vi "Channel Info.vi"(8 "error in":errorcluster, 11 "Input Channels in":refnum<class "Input Channels.lvclass">) -> (0 "error out":errorcluster, 1 "Channel Active?":bool, 2 "Channel Information":T1={"Channel Direction"=enum."Module Output", "Alias"="", "Refresh (ms)"=1000.0, "Scaling Information"={"Active"=FALSE, "Scaling Type"=enum."Linear", "Output Minimum"=0.0, "Output Maximum"=1.0, "Raw Minimum"=0.0, "Raw Maximum"=1.0, "Output Unit"="", "Function"="", "Lookup Table"=""}, "Value Type"=enum."double", "Subchannels"=[], "Auxiliary Data"=variant, "Group"=-1}, 3 "Input Channels out":refnum<class "Input Channels.lvclass">)   [LabVIEW 2020, in "Plugin.lvlib" / "Input Channels.lvclass"]
doc: "Reads the input channel data and updates the channel information cluster."
uses:
  Input Channels.lvclass
  C:/SVN_LabSys/labsys_lvcode/LabSys_SourceCode/Plugin Template/Source/Code/Channels/Plugin_Channels.lvclass
  builds/Libraries/LabSys Framework.lvlibp/Configuration Storage/Test Configuration/Channel Information.ctl
  builds/Libraries/LabSys Framework.lvlibp/Configuration Storage/Test Configuration/Channel Directions.ctl
  builds/Libraries/LabSys Framework.lvlibp/Configuration Storage/Test Configuration/Scaling Information.ctl
  builds/Libraries/LabSys Framework.lvlibp/Configuration Storage/Test Configuration/Scaling Types.ctl
  builds/Libraries/Framework Base Library.lvlibp/Value Types.ctl
  builds/Libraries/LabSys Framework.lvlibp/Configuration Storage/Test Configuration/Subchannel Information.ctl
  Typedefs/Channel Type.ctl
  UI_Class/Auxiliary Data.ctl
  Plugin_Channels.lvclass
  builds/Libraries/Framework Base Library.lvlibp
  builds/Libraries/LabSys Framework.lvlibp/Configuration Storage/Test Configuration/Test Configuration.lvclass
  UI_Class/Plugin_UI.lvclass
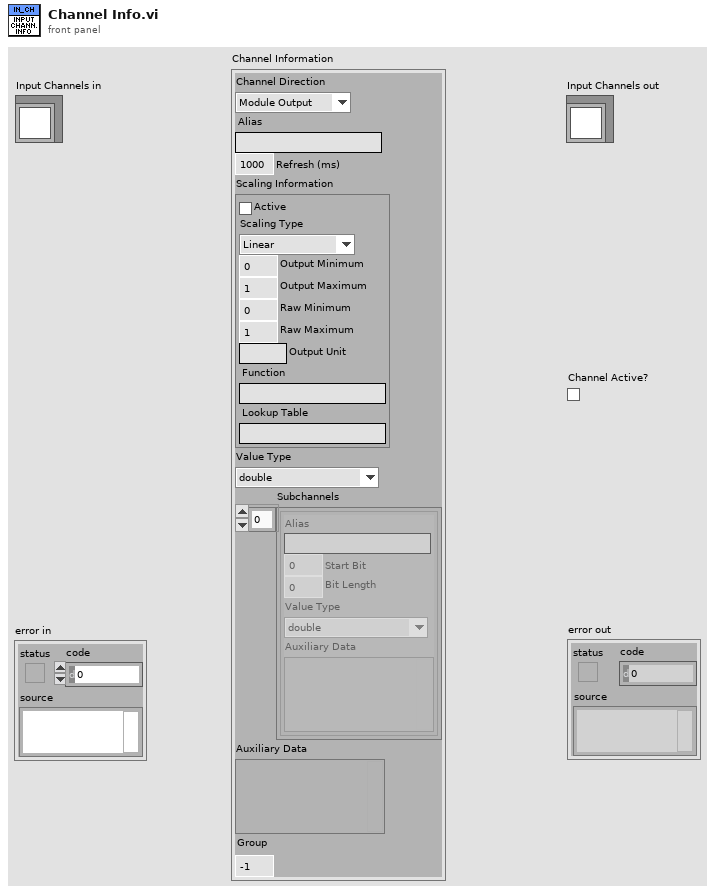
[diagram p1: front panel]
types:
  T1 = typedef "LabSys Framework.lvlibp/Configuration Storage.lvlib/Test Configuration.lvclass/Channel Information.ctl" = cluster{"Channel Direction":T2, "Alias":string, "Refresh (ms)":dbl, "Scaling Information":T3, "Value Type":T5, "Subchannels":T6[], "Auxiliary Data":variant, "Group":i32}
  T2 = typedef "LabSys Framework.lvlibp/Configuration Storage.lvlib/Test Configuration.lvclass/Channel Directions.ctl" = enum8{"Module Input", "Module Output"}
  T3 = typedef "LabSys Framework.lvlibp/Configuration Storage.lvlib/Test Configuration.lvclass/Scaling Information.ctl" = cluster{"Active":bool, "Scaling Type":T4, "Output Minimum":dbl, "Output Maximum":dbl, "Raw Minimum":dbl, "Raw Maximum":dbl, "Output Unit":string, "Function":string, "Lookup Table":string}
  T4 = typedef "LabSys Framework.lvlibp/Configuration Storage.lvlib/Test Configuration.lvclass/Scaling Types.ctl" = enum8{"Linear", "Function", "Lookup Table"}
  T5 = typedef "Framework Base Library.lvlibp/Value Types.ctl" = enum8{"Unknown", "double", "double array", "Waveform", "DigWaveform", "Boolean", "Decimal", "String", "Db2Message", "Byte Array", "Unsigned Decimal"}
  T6 = typedef "LabSys Framework.lvlibp/Configuration Storage.lvlib/Test Configuration.lvclass/Subchannel Information.ctl" = cluster{"Alias":string, "Start Bit":u32, "Bit Length":u32, "Value Type":T5, "Auxiliary Data":variant}
  T7 = typedef "Plugin.lvlib/Plugin_UI.lvclass/Auxiliary Data.ctl" = cluster{"Plugin_Data":refnum<class "Plugin_Channels.lvclass">}
  T8 = typedef "Plugin.lvlib/Plugin_Channels.lvclass/Channel Type.ctl" = enum16{"Input", "Output"}
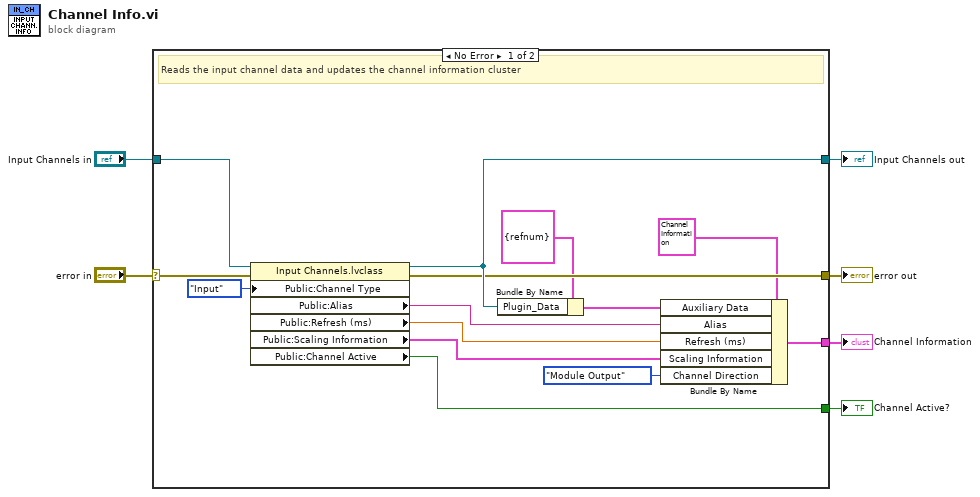
[diagram p0: block diagram]
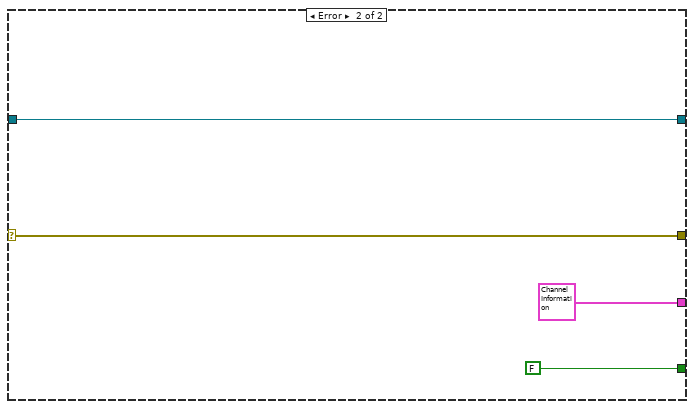
[diagram p2: hidden frame]
diagram:
  n1 = case shown="No Error" "error in" {
    selector: "error in" -> [w20 w24]
    tunnel: [w15 w24] -> w5
    tunnel: [w16 w23] -> w3
    tunnel: "Input Channels in" -> [w17 w23]
    tunnel: [w11 FALSE ("Public:Channel Active")] -> w2
    tunnel: [w10 T1 {"Channel Direction"=enum."Module Output", "Alias"="", "Refresh (ms)"=1000.0, "Scaling Information"={"Active"=FALSE, "Scaling Type"=enum."Linear", "Output Minimum"=0.0, "Output Maximum"=1.0, "Raw Minimum"=0.0, "Raw Maximum"=1.0, "Output Unit"="", "Function"="", "Lookup Table"=""}, "Value Type"=enum."double", "Subchannels"=[], "Auxiliary Data"=variant, "Group"=-1} ("Channel Information")] -> w1
    frame No Error {
      # "Reads the input channel data and updates the channel information cluster"
      n2 = property class="Input Channels.lvclass"(reference=w17, error in=w20, "Public:Channel Type"=Channel_Type."Input" ("Channel Type")) -> (reference out=w16:refnum<class "Input Channels.lvclass">, error out=w15:errorcluster, "Public:Alias"=w14:string, "Public:Refresh (ms)"=w13:dbl, "Public:Scaling Information"=w12:T3, "Public:Channel Active"=w11:bool)
      n3 = Bundle By Name(cluster=T7 {"Plugin_Data"=refnum} ("Auxiliary Data"), "Plugin_Data"=w16) -> (w18:T7)
      n4 = Bundle By Name(cluster=T1 {"Channel Direction"=enum."Module Output", "Alias"="", "Refresh (ms)"=1000.0, "Scaling Information"={"Active"=FALSE, "Scaling Type"=enum."Linear", "Output Minimum"=0.0, "Output Maximum"=1.0, "Raw Minimum"=0.0, "Raw Maximum"=1.0, "Output Unit"="", "Function"="", "Lookup Table"=""}, "Value Type"=enum."double", "Subchannels"=[], "Auxiliary Data"=variant, "Group"=-1} ("Channel Information"), "Auxiliary Data"=w18, "Alias"=w14, "Refresh (ms)"=w13, "Scaling Information"=w12, "Channel Direction"=Channel_Directions."Module Output") -> (w10:T1)
    }
    frame Error {
    }
  }
  "error out" <- w5
  "Input Channels out" <- w3
  "Channel Active?" <- w2
  "Channel Information" <- w1
